vi "ZLIB Get Current File Info__ogtk.vi"(8 "error in (no error)":errorcluster, 11 "unzip Refnum":T2) -> (0 "error out":errorcluster, 1 "file info":T1 {"file timestamp" format="%<%H:%M:%S\n%d/%m/%Y>T"; "external fa" format="%.0x"; "internal fa" format="%.0x"; "crc" format="%.0x"}, 2 "name":string, 3 "unzip Refnum out":T2)   [LabVIEW 2014, in "ZLIB.lvlib"]
doc: "Gets the info of the current file in an archive in an unzip session."
uses:
  ZLIB.lvlib
  ZLIB Unzip Handle__ogtk.ctl
  ZLIB File Info__ogtk.ctl
  ZLIB Uncompress File Info__ogtk.ctl
  lvzlib.dll
panel:
  # "Please visit http://www.OpenG.org to learn about the\nOpen Source LabVIEW software movement.\n\nNOTICE -- YOU MUST LEAVE THIS NOTICE IN PLACE.  PER THE TERMS OF THE LICENSE BELOW, YOU MAY SUBLICENSE THIS SOFTWARE \nIN ANY WAY THAT DOES NOT CONFLICT WITH THIS LICENSE.\n\n### BSD License (http://www.opensource.org/licenses/bsd-license.php) Begin ###\n \nCopyright (C) 2002-2004 Rolf Kalbermatter rolf.kalbermatter@citeng.com\nCopyright (C) 2002 Jim Kring jim@jimkring.com\n\nAll rights reserved.\n\nRedistribution and use in source and binary forms, with or without modification, are permitted provided that the following conditions are met:\n\n    * Redistributions of source code must retain the above copyright notice, this list of conditions and the following disclaimer.\n    * Redistributions in binary form must reproduce the above copyright notice, this list of conditions and the following disclaimer in the \n       documentation and/or other materials provided with the distribution.\n    * Neither the name of SciWare, James Kring, Inc., nor the names of its contributors may be used to endorse or promote products derived \n       from this software without specific prior written permission.\n\nTHIS SOFTWARE IS PROVIDED BY THE COPYRIGHT HOLDERS AND CONTRIBUTORS \"AS IS\" AND ANY EXPRESS OR IMPLIED WARRANTIES, \nINCLUDING, BUT NOT LIMITED TO, THE IMPLIED WARRANTIES OF MERCHANTABILITY AND FITNESS FOR A PARTICULAR PURPOSE ARE \nDISCLAIMED. IN NO EVENT SHALL THE COPYRIGHT OWNER OR CONTRIBUTORS BE LIABLE FOR ANY DIRECT, INDIRECT, INCIDENTAL,\n SPECIAL, EXEMPLARY, OR CONSEQUENTIAL DAMAGES (INCLUDING, BUT NOT LIMITED TO, PROCUREMENT OF SUBSTITUTE GOODS OR \nSERVICES; LOSS OF USE, DATA, OR PROFITS; OR BUSINESS INTERRUPTION) HOWEVER CAUSED AND ON ANY THEORY OF LIABILITY, \nWHETHER IN CONTRACT, STRICT LIABILITY, OR TORT (INCLUDING NEGLIGENCE OR OTHERWISE) ARISING IN ANY WAY OUT OF THE USE \nOF THIS SOFTWARE, EVEN IF ADVISED OF THE POSSIBILITY OF SUCH DAMAGE.\n\n### BSD License End ###"
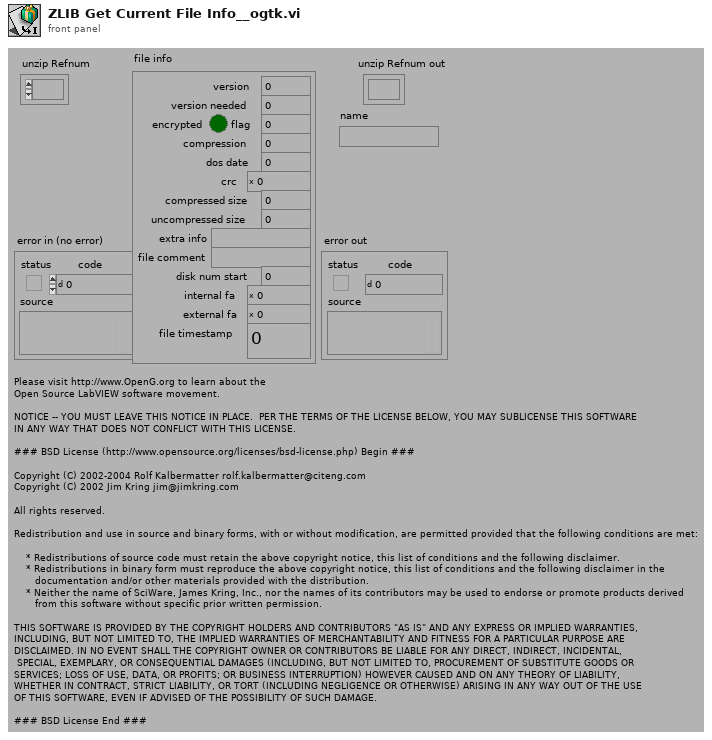
[diagram p1: front panel]
types:
  T1 = typedef "ZLIB.lvlib/ZLIB File Info__ogtk.ctl" = cluster{"version":u32, "version needed":u32, "encrypted":bool, "flag":u32, "compression":i32, "dos date":u32, "crc":u32, "compressed size":u32, "uncompressed size":u32, "extra info":string, "file comment":string, "disk num start":u32, "internal fa":u32, "external fa":u32, "file timestamp":u32}
  T2 = typedef "ZLIB.lvlib/ZLIB Unzip Handle__ogtk.ctl" = refnum<k1>
  T3 = typedef "ZLIB.lvlib/ZLIB Uncompress File Info__ogtk.ctl" = cluster{"version":u32, "version needed":u32, "flag":u32, "compression":u32, "dos date":u32, "crc":u32, "compressed size":u32, "uncompressed size":u32, "size filename":u32, "size file extra":u32, "size file comment":u32, "disk num start":u32, "internal fa":u32, "external fa":u32, "date time":cluster{"sec":i32, "min":i32, "hour":i32, "mday":i32, "mon":i32, "year":i32}}
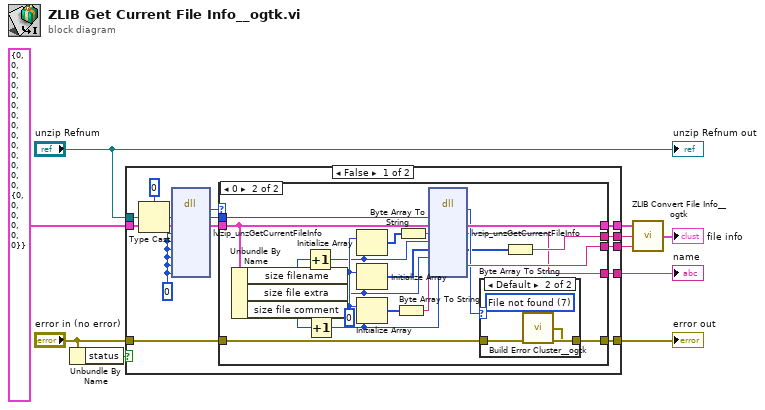
[diagram p0: block diagram]
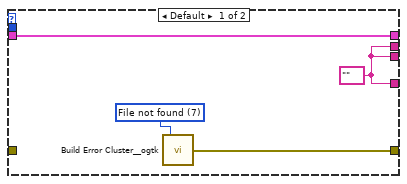
[diagram p2: hidden frame]
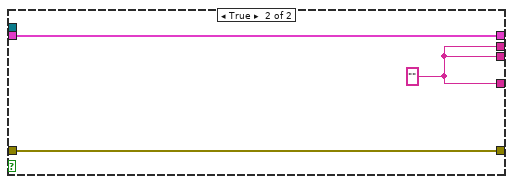
[diagram p4: hidden frame]
diagram:
  n1 = Unbundle By Name("error in (no error)") -> ("status"=w10:bool)
  n2 = case shown="False" w10 {
    tunnel: "error in (no error)" -> [w23 w54]
    tunnel: [w22 w54] -> w7
    tunnel: "unzip Refnum" -> [w20 _]
    tunnel: T3 {"version"=0, "version needed"=0, "flag"=0, "compression"=0, "dos date"=0, "crc"=0, "compressed size"=0, "uncompressed size"=0, "size filename"=0, "size file extra"=0, "size file comment"=0, "disk num start"=0, "internal fa"=0, "external fa"=0, "date time"={"sec"=0, "min"=0, "hour"=0, "mday"=0, "mon"=0, "year"=0}} ("file info") -> [w18 w52]
    tunnel: [w11 w52] -> w5
    tunnel: [w14 w53] -> w4
    tunnel: [w13 w53] -> w3
    tunnel: [w12 w53] -> w1
    frame False {
      w16 = u32 0 ("fileName")
      n3 = Type Cast(type=u32 0 ("unzFile"), x=w20) -> (*(type *) &x=w19:u32)
      n4 = dll-call lib="C:/Users/Public/SSDC/OpenDocument/LabVIEWODFToolkit/Sourcecode/SubVIs/ZLIB/lvzlib.*" fn="lvzip_unzGetCurrentFileInfo"("unzFile"=w19, "file info"=w18, "fileName"=w16, "fileNameLen"=w16, "extraField"=w16, "extraFieldLen"=w16, "comment"=w16, "commentLen"=w16) -> (w24:i32, "unzFile"=w15:u32, "file info"=w17:T3)  [unwired: 9 in, 2 out]
      n5 = case shown="0" w24 {
        tunnel: w23 -> [_ w32]
        tunnel: [w28 w32] -> w22
        tunnel: w17 -> [w26 w47]
        tunnel: w15 -> [_ w48]
        tunnel: [w26 w41] -> w11
        tunnel: [w25 w29] -> w14
        tunnel: [w25 w34] -> w13
        tunnel: [w25 w30] -> w12
        frame Default {
          w25 = "" ("fileName")
          w27 = 7 items=["No error", "Argument error", "Memory is full", "Out of zone", "End of file", "File already open", "Generic file I/O error", "File not found", "File permission error", "Disk is full", "Duplicate path", "Too many files open", "System feature not enabled", "Resource file not found", "Cannot add resource", "Resource not found", "Image not found", "Image memory error", "Pen does not exist", "Config type invalid", "Config token not found", "Config parse error", "Config memory error", "Bad external code format", "Bad external code offset", "External code not present", "Null window", "Destroy window error", "Null menu", "Print aborted", "Bad print record", "Print driver error", "Windows error during printing", "Memory error during printing", "Print dialog error", "Generic print error", "Invalid device refnum", "Device not found", "Device parameter error", "Device unit error", "Cannot open device", "Device call aborted", "Generic error", "Cancelled by user", "Object ID too low", "Object ID too high", "Object not in heap", "Unknown heap", "Unknown object (invalid DefProc)", "Unknown object (DefProc not in table)", "Message out of range", "Invalid (null) method", "Unknown message", "Manager call not supported", "Bad address", "Network operation in progress", "Network operation timed out", "Connection is busy", "Network attribute not supported", "Network error", "Address in use", "System out of memory", "Connection aborted", "Connection refused", "Not connected", "Already connected", "Connection closed", "Initialization error (interapplication manager)", "Bad occurrence", "Wait on unbound occurrence handler", "Occurrence queue overflow", "Datalog type conflict", "Unused", "Unrecognized type (interapplication manager)", "Memory corrupt", "Failed to make temporary DLL", "Old CIN version", "Drag socket not found", "Failed to load drop-object", "Failed to register OLE object", "Failed to release OLE object", "Format specifier type mismatch", "Unknown format specifier", "Too few format specifiers", "Too many format specifiers", "Scan failed", "Newer CIN version", "Error converting to variant", "Runtime menu error", "Password tampered", "Variant attribute not found", "Incompatible variant data type", "Event data is not available", "Event Store is not present", "Occurrence is not found", "Event Queue is not created", "Event info is not available", "Refnum passed is NULL", "Error retrieving Class GUID", "Error retrieving CoClass GUID", "Error retrieving TypeLib GUID.", "Bad built application magic bytes.", "Specific driver is different from the specific driver associated with the Logical Name.", "There is no session opened to the class driver.", "Max Error", "MAX - Error with config objects", "MAX - Error loading configuration", "MAX - Group not supported"]
          n6 = call "Build Error Cluster__ogtk.vi"("code"=w27) -> ("error out"=w28:errorcluster)  [unwired: 1 in]
        }
        frame 0 {
          w44 = u8 0
          n7 = Unbundle By Name(w47) -> ("size filename"=w46:u32, "size file extra"=w35:u32, "size file comment"=w45:u32)
          n8 = Increment(x=w46) -> (x+1=w43:u32)
          n9 = Increment(x=w45) -> (x+1=w42:u32)
          n10 = Initialize Array(w44, w43) -> (w40:u8[])
          n11 = Initialize Array(w44, w35) -> (w38:u8[])
          n12 = Initialize Array(w44, w42) -> (w37:u8[])
          n13 = Byte Array To String(unsigned byte array=w37) -> (string=w36:string)
          n14 = Byte Array To String(unsigned byte array=w40) -> (string=w39:string)
          n15 = dll-call lib="C:/Users/Public/SSDC/OpenDocument/LabVIEWODFToolkit/Sourcecode/SubVIs/ZLIB/lvzlib.*" fn="lvzip_unzGetCurrentFileInfo"("unzFile"=w48, "file info"=w47, "fileName"=w39, "fileNameLen"=w43, "extraField"=w38, "extraFieldLen"=w35, "comment"=w36, "commentLen"=w42) -> (w33:i32, "file info"=w41:T3, "fileName"=w29:string, "extraField"=w31:u8[], "comment"=w34:string)  [unwired: 7 in, 2 out]
          n16 = case shown="Default" w33 {
            tunnel: w32 -> [w49 _]
            tunnel: [w49 w50] -> _
            frame 0 {
            }
            frame Default {
              w51 = 7 items=["No error", "Argument error", "Memory is full", "Out of zone", "End of file", "File already open", "Generic file I/O error", "File not found", "File permission error", "Disk is full", "Duplicate path", "Too many files open", "System feature not enabled", "Resource file not found", "Cannot add resource", "Resource not found", "Image not found", "Image memory error", "Pen does not exist", "Config type invalid", "Config token not found", "Config parse error", "Config memory error", "Bad external code format", "Bad external code offset", "External code not present", "Null window", "Destroy window error", "Null menu", "Print aborted", "Bad print record", "Print driver error", "Windows error during printing", "Memory error during printing", "Print dialog error", "Generic print error", "Invalid device refnum", "Device not found", "Device parameter error", "Device unit error", "Cannot open device", "Device call aborted", "Generic error", "Cancelled by user", "Object ID too low", "Object ID too high", "Object not in heap", "Unknown heap", "Unknown object (invalid DefProc)", "Unknown object (DefProc not in table)", "Message out of range", "Invalid (null) method", "Unknown message", "Manager call not supported", "Bad address", "Network operation in progress", "Network operation timed out", "Connection is busy", "Network attribute not supported", "Network error", "Address in use", "System out of memory", "Connection aborted", "Connection refused", "Not connected", "Already connected", "Connection closed", "Initialization error (interapplication manager)", "Bad occurrence", "Wait on unbound occurrence handler", "Occurrence queue overflow", "Datalog type conflict", "Unused", "Unrecognized type (interapplication manager)", "Memory corrupt", "Failed to make temporary DLL", "Old CIN version", "Drag socket not found", "Failed to load drop-object", "Failed to register OLE object", "Failed to release OLE object", "Format specifier type mismatch", "Unknown format specifier", "Too few format specifiers", "Too many format specifiers", "Scan failed", "Newer CIN version", "Error converting to variant", "Runtime menu error", "Password tampered", "Variant attribute not found", "Incompatible variant data type", "Event data is not available", "Event Store is not present", "Occurrence is not found", "Event Queue is not created", "Event info is not available", "Refnum passed is NULL", "Error retrieving Class GUID", "Error retrieving CoClass GUID", "Error retrieving TypeLib GUID.", "Bad built application magic bytes.", "Specific driver is different from the specific driver associated with the Logical Name.", "There is no session opened to the class driver.", "Max Error", "MAX - Error with config objects", "MAX - Error loading configuration", "MAX - Group not supported"]
              n17 = call "Build Error Cluster__ogtk.vi"("code"=w51) -> ("error out"=w50:errorcluster)  [unwired: 1 in]
            }
          }
          n18 = Byte Array To String(unsigned byte array=w31) -> (string=w30:string)
        }
      }
    }
    frame True {
      w53 = "" ("fileName")
    }
  }
  "error out" <- w7
  "name" <- w4
  n19 = call "ZLIB Convert File Info__ogtk.vi"("comment"=w3, "extra field"=w1, "uncompress file info in"=w5) -> ("file info out"=→"file info":T1)
  "unzip Refnum out" <- "unzip Refnum"
